vi "Teleop.vi"(10 "Match Info":T1={"Autonomous Elapsed Seconds"=0.0, "TeleOp Elapsed Seconds"=0.0, "Disabled Elapsed Seconds"=0.0, "Visited Autonomous"=FALSE, "Visited TeleOp"=FALSE, "Visited Disabled"=FALSE, "Autonomous Settings"={"Autonomous Style"=enum."Independent", "VI Refnum"=refnum}}, 11 "Call Context":T2) -> ()   [LabVIEW 2019]
doc: "This VI is called for each TeleOp packet received from the DS where the robot is not disabled. It is often used to read from the joysticks and update I/O or to update setpoints for timed control loops. It should complete and return within 20 milliseconds or it may miss DS packets."
uses:
  <vilib>/Rock Robotics/WPI/DriverStation/WPI_DriverStationDerivedRobotMode.ctl
  <vilib>/Rock Robotics/WPI/DriverStation/WPI_DriverStationMatch Info.ctl
  Functions/Global Variables/Robot State.vi
  Functions/Global Variables/Trajectory Enabled.vi
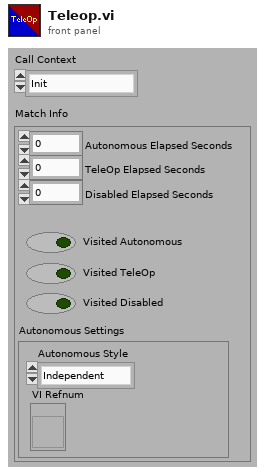
[diagram p1: front panel]
types:
  T1 = typedef "WPI_DriverStationMatch Info.ctl" = cluster{"Autonomous Elapsed Seconds":dbl, "TeleOp Elapsed Seconds":dbl, "Disabled Elapsed Seconds":dbl, "Visited Autonomous":bool, "Visited TeleOp":bool, "Visited Disabled":bool, "Autonomous Settings":cluster{"Autonomous Style":enum16{"Iterative", "Independent"}, "VI Refnum":refnum<vi>}}
  T2 = typedef "WPI_DriverStationDerivedRobotMode.ctl" = enum16{"Init", "Execute", "Stop"}
  T3 = typedef "Robot State.ctl" = cluster{"Drive System State":T4, "Enable Actions":T7, "Lift System Actions":T8, "SpinnerActions":T9, "Ball System Actions":T10}
  T4 = typedef "Robot Pivot Motion Commands.ctl" = cluster{"Front Right":T5, "Front Left":T5, "Rear Left":T5, "Rear Right":T5, "Drive Mode":T6, "Reset Drive Encoder":bool}
  T5 = typedef "Pivot Motor Commands.ctl" = cluster{"Drive Power":dbl, "Drive Distance (in)":dbl, "Drive Distance Error (in)":dbl, "Steer Power":dbl, "Steer Angle (deg)":dbl, "Steer Angle Error (deg)":dbl}
  T6 = typedef "Robot Drive Mode.ctl" = enum16{"Velocity", "Distance"}
  T7 = typedef "Enable Actions.ctl" = cluster{"Swerve Drive":bool, "Color System":bool, "Ball System":bool, "Lift System":bool}
  T8 = typedef "Lift System Actions.ctl" = cluster{"Arm Deploy Piston":bool, "Enable Lift Arm":bool, "Enable Climber":bool, "Climber Velocity":dbl, "Lift Arm Velocity":dbl}
  T9 = typedef "Spinner Actions.ctl" = cluster{"Manual Mode ":bool, "Auto rotate n times":bool, "Auto rotate to color\t":bool, "Extend and Retract Arm\t":bool, "Manual Rotation Speed":dbl}
  T10 = typedef "Ball System Actions.ctl" = cluster{"Intake Piston ":bool, "Shoot Ball":bool, "Tube up one Increment\t":bool, "Reverse Ball Intake":bool, "Tube Piston":bool, "Enable Manual Tube":bool, "Tube up four Increments":bool, "Manual Tube Velocity":dbl, "Ball Intake Speed":dbl}
  T11 = typedef "DriveJoystickData.ctl" = cluster{"Relative Encoders?":bool, "Zero Steer Encoder":bool, "Reset Field Orientation":bool, "Use Field Orientation":bool, "Drive X":dbl, "Drive Y":dbl, "Drive Z":dbl, "Fast Speed Accelerator":dbl, "Increase Max Speed":bool, "Decrease Max Speed":bool, "Camera Controller":bool}
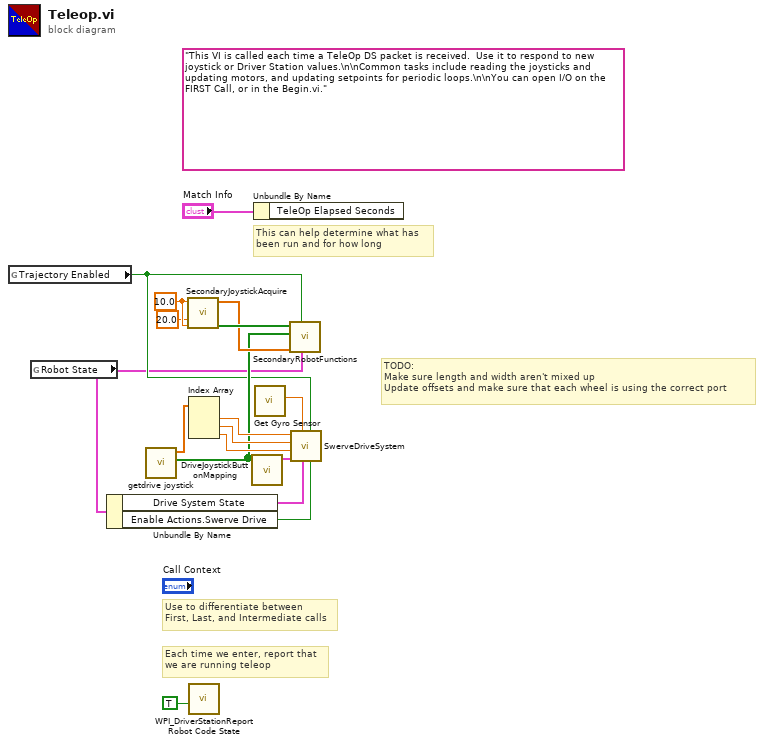
[diagram p0: block diagram]
diagram:
  w13 = 10.0 ("XY Joystick Deadband %")
  (unwired) "This VI is called each time a TeleOp DS packet is received.  Use it to respond to new joystick or Driver Station values.\n\nCommon tasks include reading the joysticks and updating motors, and updating setpoints for periodic loops.\n\nYou can open I/O on the FIRST Call, or in the Begin.vi."
  # "TODO:\nMake sure length and width aren't mixed up\nUpdate offsets and make sure that each wheel is using the correct port"
  # "Each time we enter, report that\nwe are running teleop"
  # "Use to differentiate between\nFirst, Last, and Intermediate calls"
  # "This can help determine what has\nbeen run and for how long"
  n1 = global read "Trajectory Enabled.vi" "Trajectory Enabled"() -> (w5:bool)
  n2 = global read "Robot State.vi" "Robot State"() -> (w4:T3)
  n3 = Unbundle By Name(w4) -> ("Drive System State"=w3:T4, "Enable Actions.Swerve Drive"=w2:bool)
  n4 = call "getdrive joystick.vi"() -> ("drive joystick buttons"=w6:bool[], "drive joystick values"=w10:dbl[])  [unwired: 10 in]
  n5 = call "SecondaryJoystickAcquire.vi"("Rotation Joystick Deadband %"=w13, "Y Joystick Deadband %"=20.0, "X Joystick Deadband %"=w13) -> ("Secondary Joystick Buttons"=w15:bool[], "Secondary Joystick Values"=w14:dbl[])  [unwired: 7 in]
  n6 = Index Array(array=w10) -> (element #1=w9:dbl, element #2=w8:dbl, element #3=w7:dbl)  [unwired: 3 in]
  n7 = call <vilib>:"WPI_DriverStationReport Robot Code State.vi"("TeleOp"=TRUE ("Autonomous")) -> ()  [unwired: 10 in, 1 out]
  n8 = call "DriveJoystickButtonMapping.vi"("drive joystick buttons"=w6) -> ("output cluster"=w11:T11)  [unwired: 9 in, 1 out]
  n9 = Unbundle By Name("Match Info") -> ()  [unwired: 1 out]
  n10 = call "Get Gyro Sensor.vi"() -> ("Robot Field Orientation (deg)"=w12:dbl)  [unwired: 11 in]
  n11 = call "SecondaryRobotFunctions.vi"("Robot State"=w4, "Automatic State Control Mode (F)"=w5, "Secondary Joystick Values"=w14, "Drive Joystick Buttons"=w6, "Secondary Joystick Buttons"=w15) -> ()  [unwired: 7 in]
  n12 = call "SwerveDriveSystem.vi"("Enable Auto Swerve Drive"=w2, "Automatic State Control Mode (F)"=w5, "Robot Motion Commands"=w3, "Robot field orientation (deg)"=w12, "Drive Joystick Buttons"=w11, "Turn"=w7, "Forward"=w8, "Right"=w9) -> ()  [unwired: 4 in]
